vi "GlobalGetInitialisationStatus.vi"() -> ()   [LabVIEW 2011]
panel:
  out "DeviceStartUpDone":bool
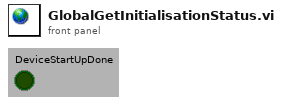
[diagram p1: front panel]
diagram:
